vi "CloseVISA.vi"(0 "object in":refnum<class "DAQ.lvclass">, 5 "error in (no error)":errorcluster) -> (14 "object out":refnum<class "DAQ.lvclass">, 19 "error out":errorcluster)   [LabVIEW 2021, in "DAQ.lvclass"]
uses:
  DAQ.lvclass
  DAQ.lvclass/DAQ.ctl
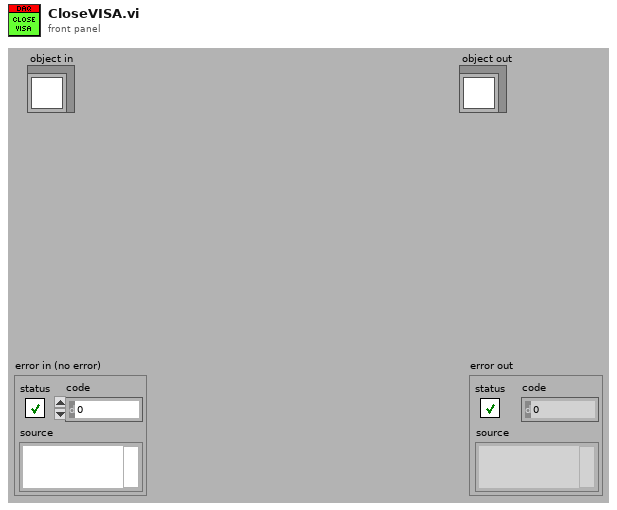
[diagram p1: front panel]
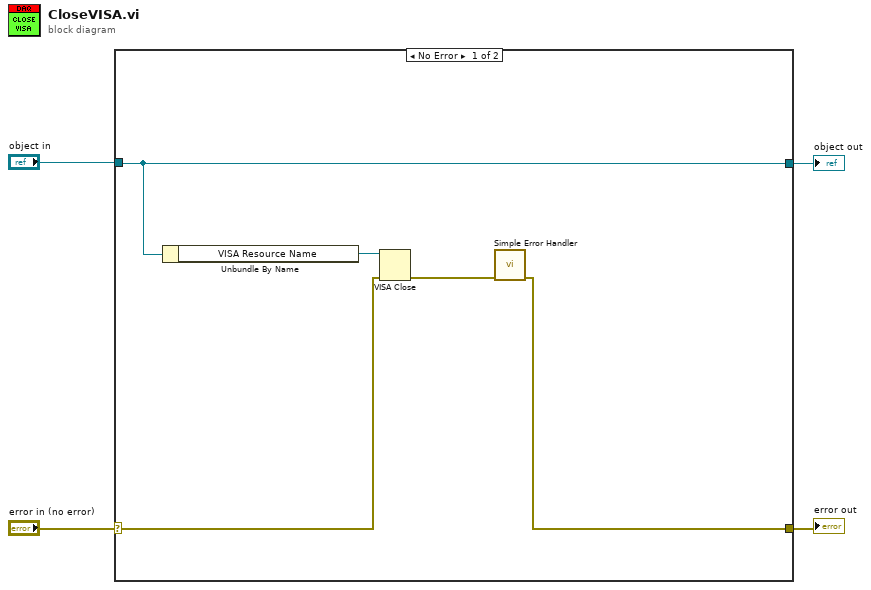
[diagram p0: block diagram]
diagram:
  n1 = case shown="No Error" "error in (no error)" {
    selector: "error in (no error)" -> [w7 w11]
    tunnel: [w5 w11] -> w3
    tunnel: [w9 w10] -> w1
    tunnel: "object in" -> [w9 w10]
    frame No Error {
      n2 = Unbundle By Name(w9) -> ("VISA Resource Name"=w8:refnum<visa-resource-name>)
      n3 = VISA Close(VISA resource name=w8, error in (no error)=w7) -> (error out=w6:errorcluster)
      n4 = call <vilib>:"Simple Error Handler.vi"("error in (no error)"=w6) -> ("error out"=w5:errorcluster)  [unwired: 4 in, 4 out]
    }
    frame Error {
    }
  }
  "error out" <- w3
  "object out" <- w1
